vi "StaticCalibration3.vi"(0 "SENSOR":T1, 11 "error in (no error)":errorcluster caption="错误输入（无错误）") -> (2 "T1(%)":dbl, 3 "T2(%)":dbl, 4 "Vres":dbl, 6 "Angle out":dbl, 8 "Vres_FD":i32, 10 "OK":bool, 13 "P(%)":dbl, 14 "S(%)":dbl, 15 "error out":errorcluster caption="错误输出")   [LabVIEW 2020]
doc: "该模板用于创建子VI。"
uses:
  <userlib>/DAQNavi Polymorphic VI/create/DAQNavi Create Channel.vi
  <userlib>/DAQNavi Polymorphic VI/create/DAQNavi Create Channel(CI-PulseWidth).vi
  <userlib>/DAQNavi Polymorphic VI/read/DAQNavi Read.vi
  <userlib>/DAQNavi Polymorphic VI/read/DAQNavi Read (Counter Pulse Width 1Chan 1Samp).vi
  <userlib>/_MGI/1D Array/MGI Average.vi
  <userlib>/_MGI/1D Array/MGI Average/MGI Average (DBL[]).vi
  <userlib>/DAQNavi Polymorphic VI/configure/task/DAQNavi Clear Task.vi
  Global_Variable/Global.vi
  <vilib>/Comparison/Less/Less Functor/Less Functor.lvclass
  <userlib>/Hella PGI/Hella PGI.lvlib
panel:
  out "T2ROC_1+T2ROC_2":i32
  out "T1ROC_1+T1ROC_2":i32
  out "PROC_1":i32
  out "T2ROC_1":i32
  out "T1ROC_1":i32
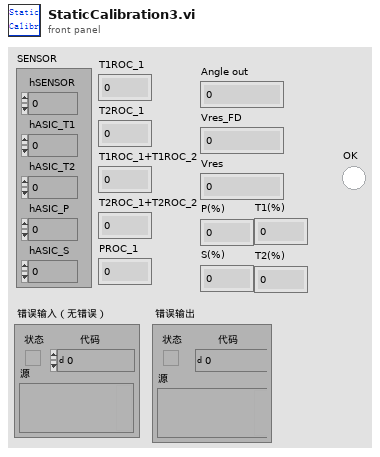
[diagram p1: front panel]
types:
  T1 = cluster{"hSENSOR":i32, "hASIC_T1":i32, "hASIC_T2":i32, "hASIC_P":i32, "hASIC_S":i32}
  T2 = cluster{"主信号":cluster{"单位":string, "下限":dbl, "上限":dbl}, "副信号":cluster{"单位":string, "下限":dbl, "上限":dbl}, "主副和":cluster{"单位":string, "下限":dbl, "上限":dbl}, "主副差":cluster{"单位":string, "下限":dbl, "上限":dbl}, "Vres":cluster{"单位":string, "下限":dbl, "上限":dbl}}
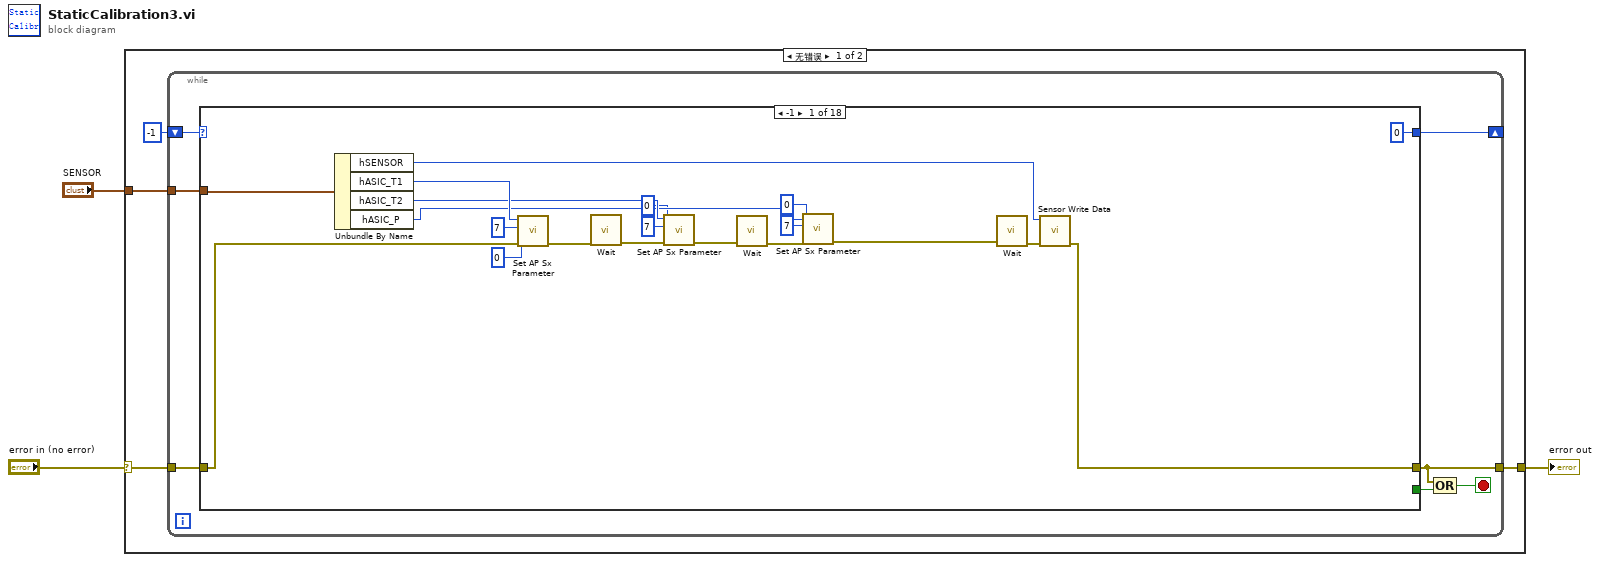
[diagram p0: block diagram]
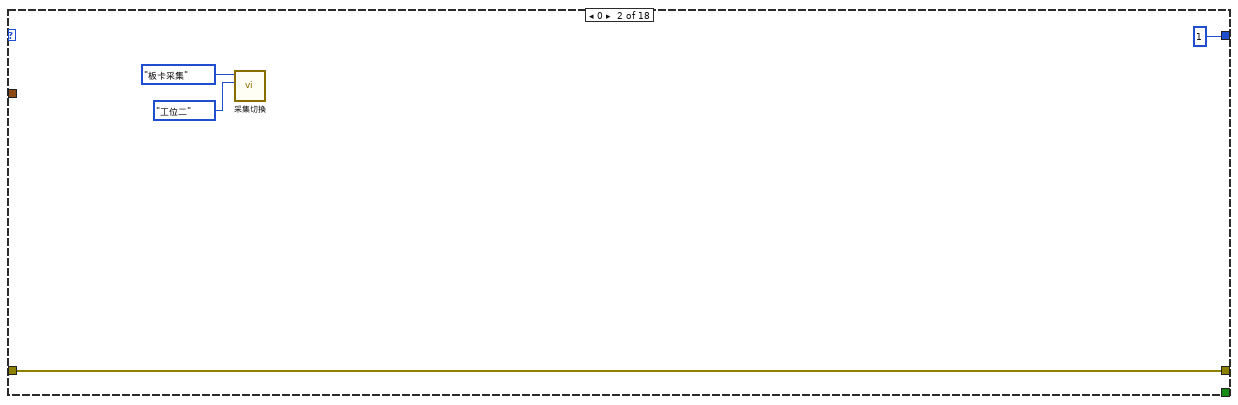
[diagram p2: hidden frame]
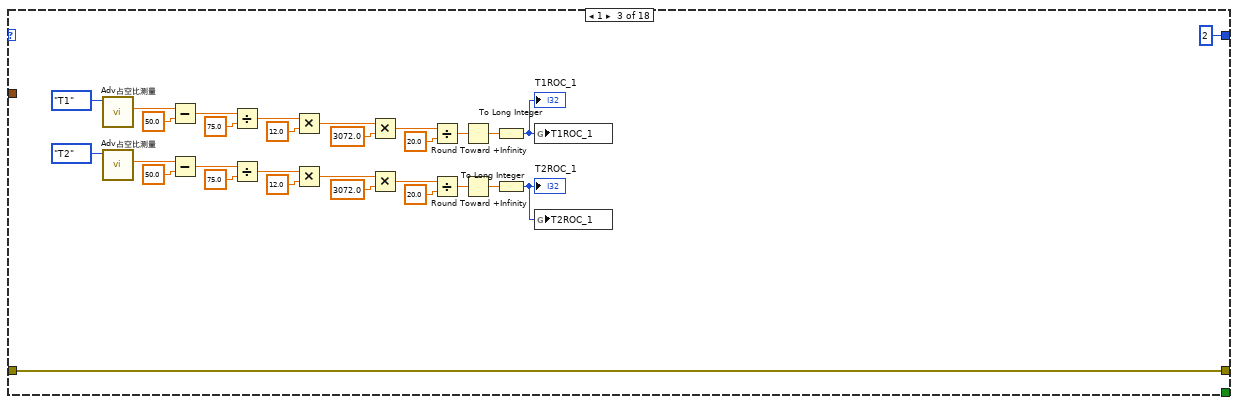
[diagram p3: hidden frame]
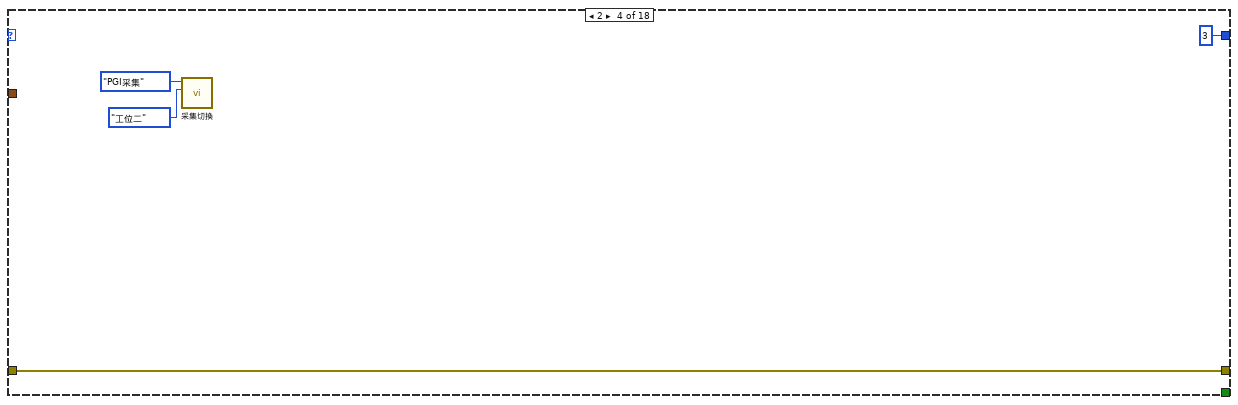
[diagram p4: hidden frame]
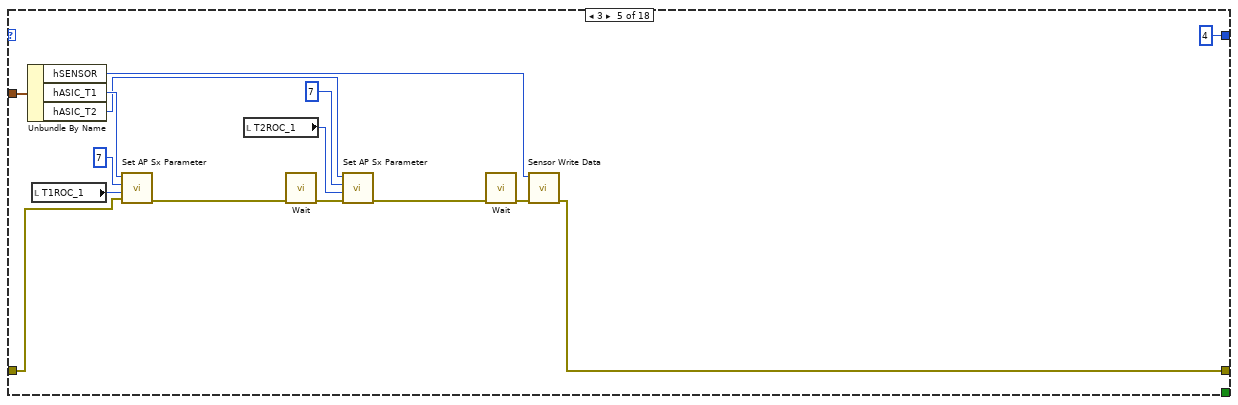
[diagram p5: hidden frame]
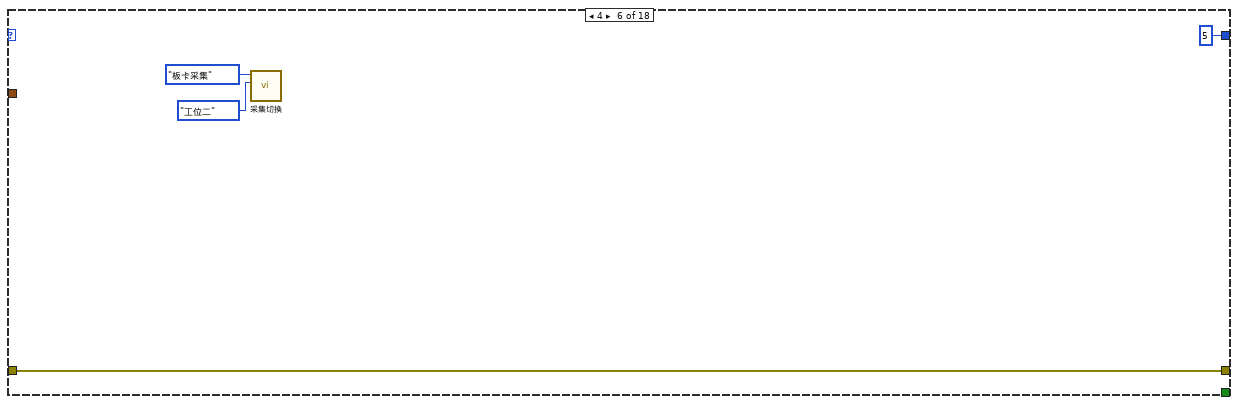
[diagram p6: hidden frame]
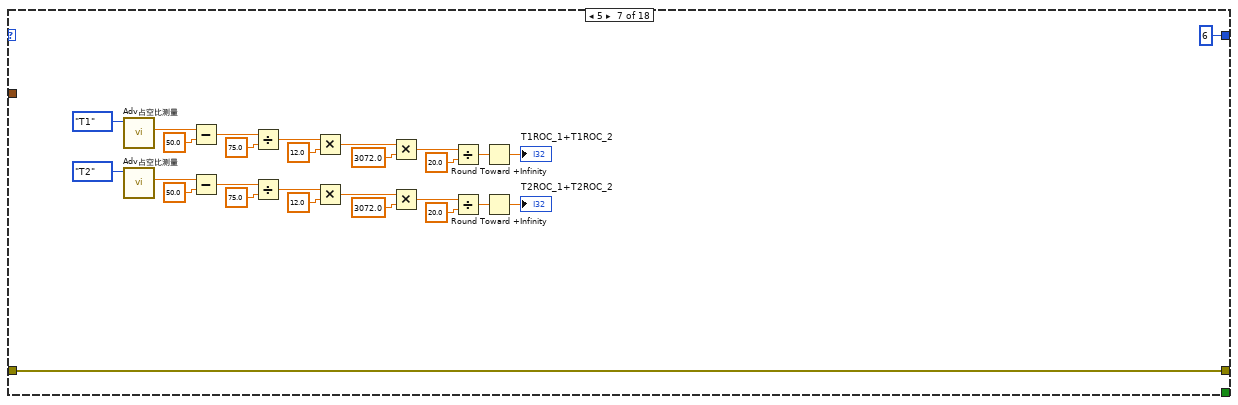
[diagram p7: hidden frame]
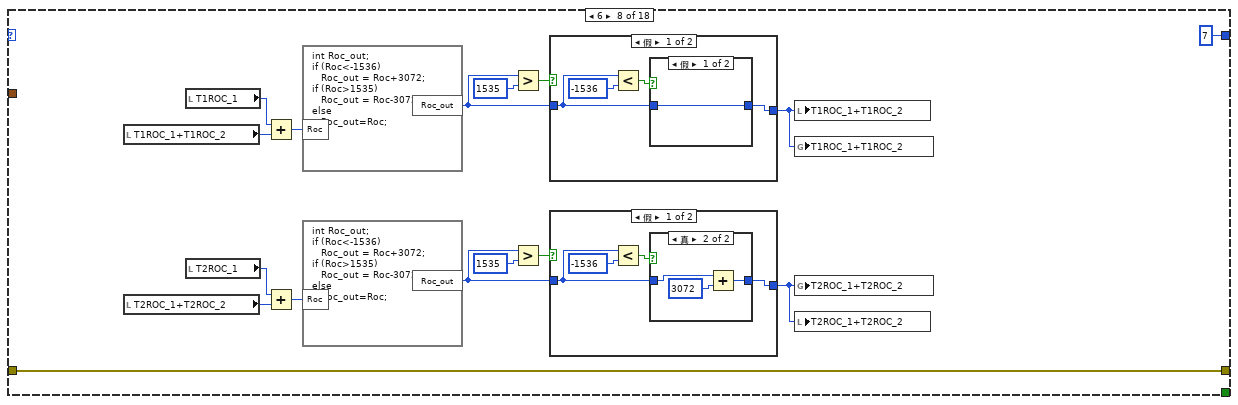
[diagram p8: hidden frame]
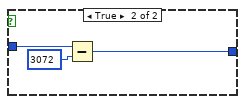
[diagram p10: hidden frame]
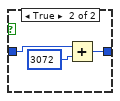
[diagram p11: hidden frame]
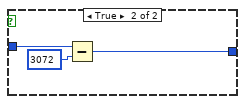
[diagram p12: hidden frame]
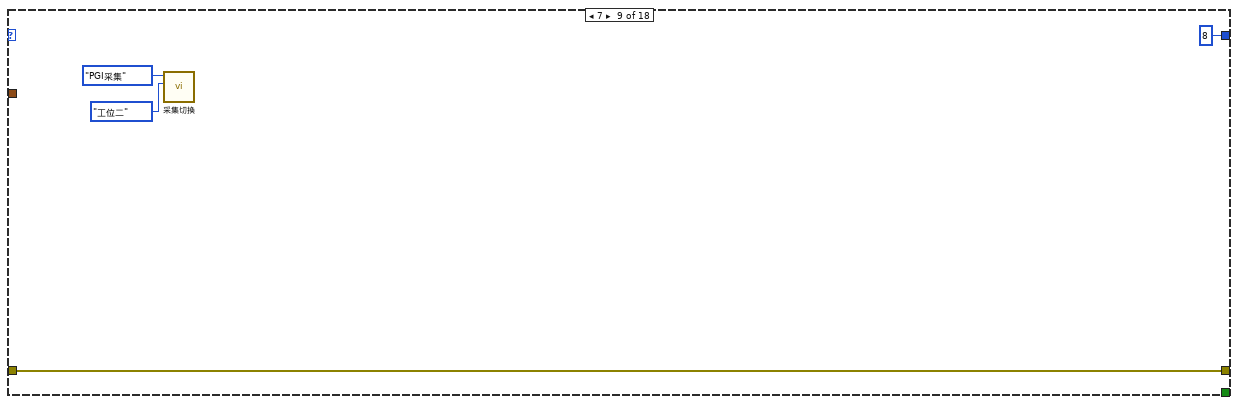
[diagram p13: hidden frame]
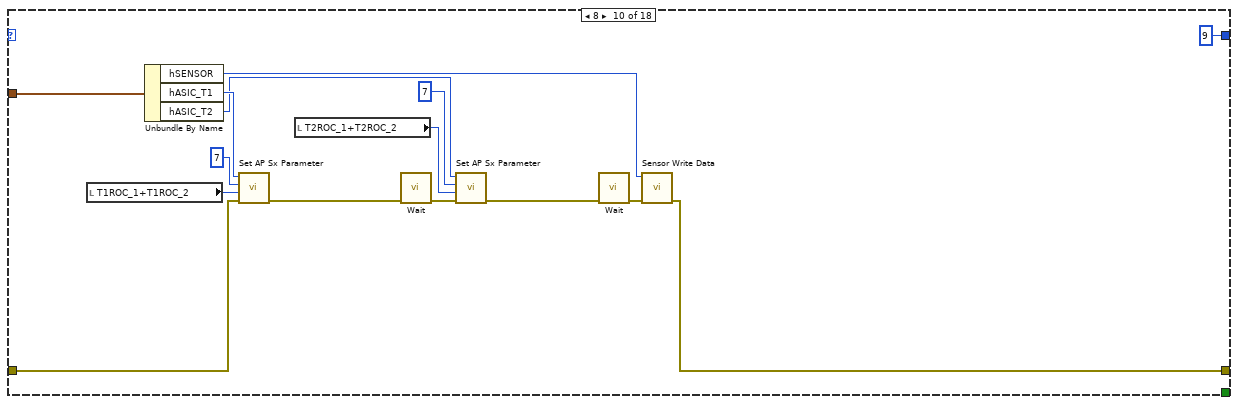
[diagram p14: hidden frame]
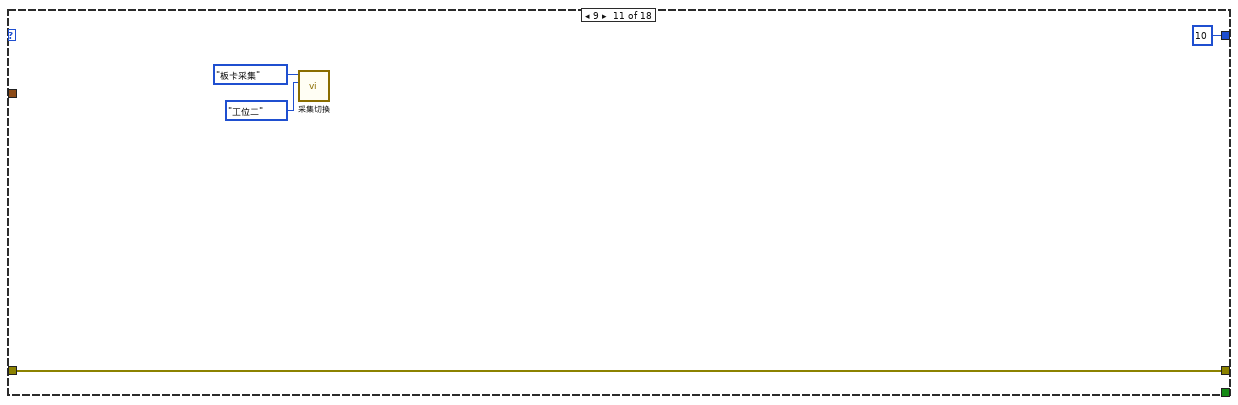
[diagram p15: hidden frame]
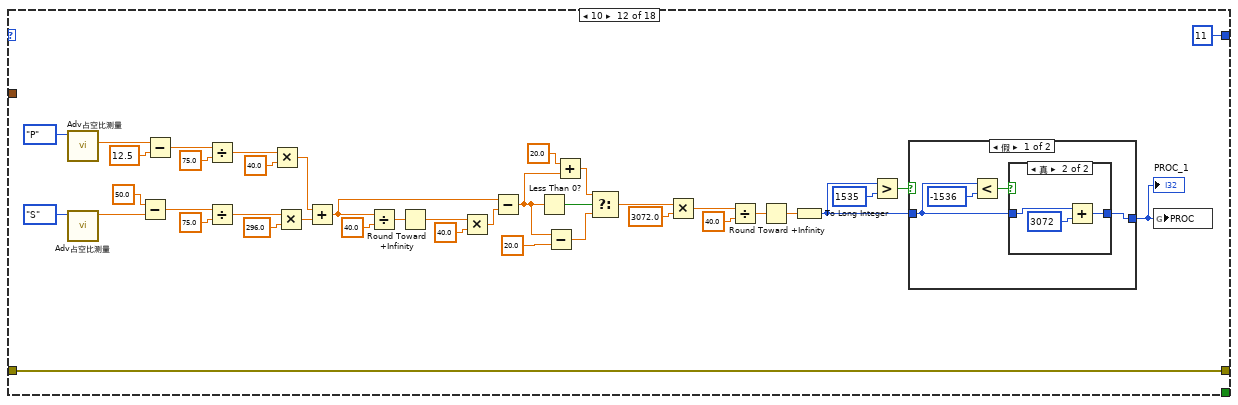
[diagram p16: hidden frame]
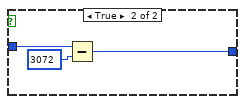
[diagram p18: hidden frame]
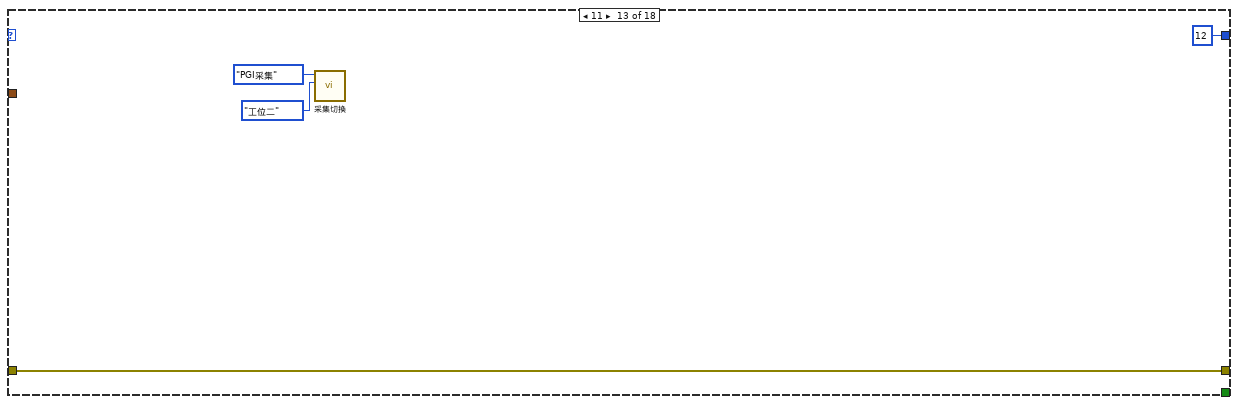
[diagram p19: hidden frame]
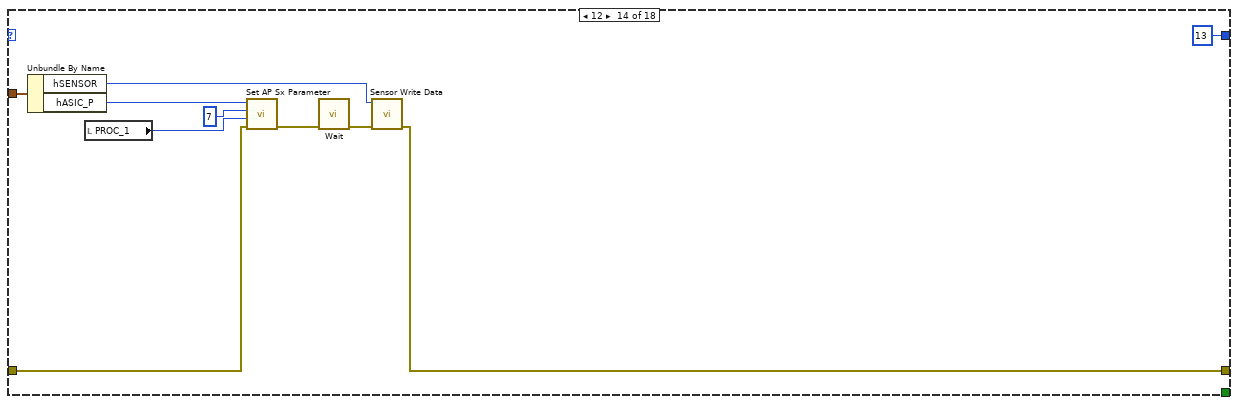
[diagram p20: hidden frame]
diagram:
  n1 = case shown="无错误" "error in (no error)" {
    selector: "error in (no error)" -> [w6 w273]
    tunnel: [w4 w273] -> w2
    tunnel: "SENSOR" -> [w7 _]
    frame No Error {
      n2 = while {
        tunnel: w7 -> [w14]
        tunnel: w6 -> [w13]
        shift-right: [w8] -> _
        shift-left: -1 -> [w12]
        tunnel: [w11] -> w4
        stop <- w10 stop-if-true
        n3 = case shown="-1" w12 {
          tunnel: w14 -> [w18 _ _ _ w85 _ _ _ _ w175 _ _ _ w241 _ _ _ _]
          tunnel: w13 -> [w17 w36 w39 w69 w79 w89 w92 w120 w158 w163 w177 w184 w232 w237 w246 w250 w264 w272]
          selector: w12 -> [_ _ _ _ _ _ _ _ _ _ _ _ _ _ _ _ _ w270]
          tunnel: [w16 w36 w39 w69 w73 w89 w92 w120 w158 w162 w177 w184 w232 w236 w246 w250 w264 w272] -> w11
          tunnel: [_ _ _ _ _ _ _ _ _ _ _ _ _ _ _ _ _ TRUE] -> w9
          tunnel: [0 1 2 3 4 5 6 7 8 9 10 11 12 13 14 15 16 w270] -> w8
          frame -1 {
            n4 = Unbundle By Name(w18) -> ("hSENSOR"=w31:i32, "hASIC_T1"=w25:i32, "hASIC_T2"=w24:i32, "hASIC_P"=w23:i32)
            n5 = call <userlib>:"Set AP Sx Parameter.vi"("error in (no error)"=w17, "para2"=0, "asicBitsName"=7, "asicHandle"=w25) -> ("error out"=w29:errorcluster)  [unwired: 6 in, 1 out]
            n6 = call "Wait.vi"("error in (no error)"=w29) -> ("error out"=w30:errorcluster)  [unwired: 6 in]
            n7 = call <userlib>:"Set AP Sx Parameter.vi"("error in (no error)"=w30, "para2"=0, "asicBitsName"=7, "asicHandle"=w24) -> ("error out"=w28:errorcluster)  [unwired: 6 in, 1 out]
            n8 = call "Wait.vi"("error in (no error)"=w28) -> ("error out"=w27:errorcluster)  [unwired: 6 in]
            n9 = call <userlib>:"Set AP Sx Parameter.vi"("error in (no error)"=w27, "para2"=0, "asicBitsName"=7, "asicHandle"=w23) -> ("error out"=w26:errorcluster)  [unwired: 6 in, 1 out]
            n10 = call "Wait.vi"("error in (no error)"=w26) -> ("error out"=w34:errorcluster)  [unwired: 6 in]
            n11 = call <userlib>:"Sensor Write Data.vi"("error in (no error)"=w34, "sensorHandle"=w31) -> ("error out"=w16:errorcluster)  [unwired: 7 in, 2 out]
          }
          frame 0 {
            n12 = call "采集切换.vi"("工位"=enum16{"工位一", "工位二"}."工位二", "采集方式"=enum16{"板卡采集", "PGI采集"}."板卡采集") -> ()  [unwired: 10 in]
          }
          frame 1 {
            n13 = call "Adv占空比测量.vi"("通道"=enum16{"T1", "T2", "P", "S"}."T1") -> ("占空比2"=w43:dbl)  [unwired: 7 in, 2 out]
            n14 = call "Adv占空比测量.vi"("通道"=enum16{"T1", "T2", "P", "S"}."T2") -> ("占空比2"=w41:dbl)  [unwired: 7 in, 2 out]
            n15 = Subtract(x=w43, y=50.0) -> (x-y=w67:dbl)
            n16 = Subtract(x=w41, y=50.0) -> (x-y=w52:dbl)
            n17 = Divide(x=w67, y=75.0) -> (x/y=w65:dbl)
            n18 = Divide(x=w52, y=75.0) -> (x/y=w54:dbl)
            n19 = Multiply(x=w65, y=12.0) -> (x*y=w63:dbl)
            n20 = Multiply(x=w54, y=12.0) -> (x*y=w56:dbl)
            n21 = Multiply(x=w63, y=3072.0) -> (x*y=w61:dbl)
            n22 = Multiply(x=w56, y=3072.0) -> (x*y=w58:dbl)
            n23 = Divide(x=w61, y=20.0) -> (x/y=w50:dbl)
            n24 = Divide(x=w58, y=20.0) -> (x/y=w49:dbl)
            n25 = Round Toward +Infinity(x=w50) -> (ceil(x): smallest int >= x=w48:dbl)
            n26 = Round Toward +Infinity(x=w49) -> (ceil(x): smallest int >= x=w47:dbl)
            n27 = To Long Integer(number=w48) -> (32bit integer=w45:i32)
            "T1ROC_1" <- w45
            n28 = To Long Integer(number=w47) -> (32bit integer=w46:i32)
            "T2ROC_1" <- w46
            n29 = global write "Global.vi" "T1ROC_1"(w45) -> ()
            n30 = global write "Global.vi" "T2ROC_1"(w46) -> ()
          }
          frame 2 {
            n31 = call "采集切换.vi"("工位"=enum16{"工位一", "工位二"}."工位二", "采集方式"=enum16{"板卡采集", "PGI采集"}."PGI采集") -> ()  [unwired: 10 in]
          }
          frame 3 {
            n32 = Unbundle By Name(w85) -> ("hSENSOR"=w82:i32, "hASIC_T1"=w84:i32, "hASIC_T2"=w83:i32)
            n33 = local read "T1ROC_1"() -> (w86:i32)
            n34 = call <userlib>:"Set AP Sx Parameter.vi"("error in (no error)"=w79, "para2"=w86, "asicBitsName"=7, "asicHandle"=w84) -> ("error out"=w78:errorcluster)  [unwired: 6 in, 1 out]
            n35 = local read "T2ROC_1"() -> (w87:i32)
            n36 = call "Wait.vi"("error in (no error)"=w78) -> ("error out"=w77:errorcluster)  [unwired: 6 in]
            n37 = call <userlib>:"Set AP Sx Parameter.vi"("error in (no error)"=w77, "para2"=w87, "asicBitsName"=7, "asicHandle"=w83) -> ("error out"=w76:errorcluster)  [unwired: 6 in, 1 out]
            n38 = call "Wait.vi"("error in (no error)"=w76) -> ("error out"=w75:errorcluster)  [unwired: 6 in]
            n39 = call <userlib>:"Sensor Write Data.vi"("error in (no error)"=w75, "sensorHandle"=w82) -> ("error out"=w73:errorcluster)  [unwired: 7 in, 2 out]
          }
          frame 4 {
            n40 = call "采集切换.vi"("工位"=enum16{"工位一", "工位二"}."工位二", "采集方式"=enum16{"板卡采集", "PGI采集"}."板卡采集") -> ()  [unwired: 10 in]
          }
          frame 5 {
            n41 = call "Adv占空比测量.vi"("通道"=enum16{"T1", "T2", "P", "S"}."T1") -> ("占空比2"=w95:dbl)  [unwired: 7 in, 2 out]
            n42 = call "Adv占空比测量.vi"("通道"=enum16{"T1", "T2", "P", "S"}."T2") -> ("占空比2"=w94:dbl)  [unwired: 7 in, 2 out]
            n43 = Subtract(x=w95, y=50.0) -> (x-y=w112:dbl)
            n44 = Subtract(x=w94, y=50.0) -> (x-y=w119:dbl)
            n45 = Divide(x=w112, y=75.0) -> (x/y=w113:dbl)
            n46 = Divide(x=w119, y=75.0) -> (x/y=w118:dbl)
            n47 = Multiply(x=w113, y=12.0) -> (x*y=w114:dbl)
            n48 = Multiply(x=w118, y=12.0) -> (x*y=w117:dbl)
            n49 = Multiply(x=w114, y=3072.0) -> (x*y=w115:dbl)
            n50 = Multiply(x=w117, y=3072.0) -> (x*y=w116:dbl)
            n51 = Divide(x=w115, y=20.0) -> (x/y=w111:dbl)
            n52 = Divide(x=w116, y=20.0) -> (x/y=w110:dbl)
            n53 = Round Toward +Infinity(x=w111) -> (ceil(x): smallest int >= x=→"T1ROC_1+T1ROC_2":dbl)
            n54 = Round Toward +Infinity(x=w110) -> (ceil(x): smallest int >= x=→"T2ROC_1+T2ROC_2":dbl)
          }
          frame 6 {
            n55 = local read "T1ROC_1+T1ROC_2"() -> (w125:i32)
            n56 = local read "T2ROC_1+T2ROC_2"() -> (w124:i32)
            n57 = local read "T1ROC_1"() -> (w133:i32)
            n58 = local read "T2ROC_1"() -> (w132:i32)
            n59 = Add(x=w133, y=w125) -> (x+y=w135:i32)
            n60 = Add(x=w132, y=w124) -> (x+y=w134:i32)
            n61 = formula code="int Roc_out;\nif (Roc<-1536)\n   Roc_out = Roc+3072;\nif (Roc>1535)\n   Roc_out = Roc-3072;\nelse\n   Roc_out=Roc;"("Roc"=w135) -> ("Roc_out"=w129:i32)
            n62 = formula code="int Roc_out;\nif (Roc<-1536)\n   Roc_out = Roc+3072;\nif (Roc>1535)\n   Roc_out = Roc-3072;\nelse\n   Roc_out=Roc;"("Roc"=w134) -> ("Roc_out"=w126:i32)
            n63 = Greater?(x=w129, y=1535) -> (0:w130:bool)
            n64 = Greater?(x=w126, y=1535) -> (0:w127:bool)
            n65 = case shown="假" w130 {
              tunnel: w129 -> [w148 w156]
              tunnel: [w147 w155] -> w123
              frame False {
                n66 = Less?(x=w148, y=-1536) -> (x < y?=w149:bool)
                n67 = case shown="假" w149 {
                  tunnel: w148 -> [w151 w154]
                  tunnel: [w151 w152] -> w147
                  frame False {
                  }
                  frame True {
                    n68 = Add(x=w154, y=3072) -> (x+y=w152:i32)
                  }
                }
              }
              frame True {
                n69 = Subtract(x=w156, y=3072) -> (x-y=w155:i32)
              }
            }
            n70 = case shown="假" w127 {
              tunnel: w126 -> [w137 w145]
              tunnel: [w136 w144] -> w122
              frame False {
                n71 = Less?(x=w137, y=-1536) -> (x < y?=w138:bool)
                n72 = case shown="真" w138 {
                  tunnel: w137 -> [w140 w143]
                  tunnel: [w140 w141] -> w136
                  frame False {
                  }
                  frame True {
                    n73 = Add(x=w143, y=3072) -> (x+y=w141:i32)
                  }
                }
              }
              frame True {
                n74 = Subtract(x=w145, y=3072) -> (x-y=w144:i32)
              }
            }
            n75 = local write "T1ROC_1+T1ROC_2"(w123) -> ()
            n76 = global write "Global.vi" "T1ROC_1+T1ROC_2"(w123) -> ()
            n77 = global write "Global.vi" "T2ROC_1+T2ROC_2"(w122) -> ()
            n78 = local write "T2ROC_1+T2ROC_2"(w122) -> ()
          }
          frame 7 {
            n79 = call "采集切换.vi"("工位"=enum16{"工位一", "工位二"}."工位二", "采集方式"=enum16{"板卡采集", "PGI采集"}."PGI采集") -> ()  [unwired: 10 in]
          }
          frame 8 {
            n80 = local read "T1ROC_1+T1ROC_2"() -> (w171:i32)
            n81 = Unbundle By Name(w175) -> ("hSENSOR"=w172:i32, "hASIC_T1"=w174:i32, "hASIC_T2"=w173:i32)
            n82 = call <userlib>:"Set AP Sx Parameter.vi"("error in (no error)"=w163, "para2"=w171, "asicBitsName"=7, "asicHandle"=w174) -> ("error out"=w168:errorcluster)  [unwired: 6 in, 1 out]
            n83 = local read "T2ROC_1+T2ROC_2"() -> (w176:i32)
            n84 = call "Wait.vi"("error in (no error)"=w168) -> ("error out"=w167:errorcluster)  [unwired: 6 in]
            n85 = call <userlib>:"Set AP Sx Parameter.vi"("error in (no error)"=w167, "para2"=w176, "asicBitsName"=7, "asicHandle"=w173) -> ("error out"=w166:errorcluster)  [unwired: 6 in, 1 out]
            n86 = call "Wait.vi"("error in (no error)"=w166) -> ("error out"=w165:errorcluster)  [unwired: 6 in]
            n87 = call <userlib>:"Sensor Write Data.vi"("error in (no error)"=w165, "sensorHandle"=w172) -> ("error out"=w162:errorcluster)  [unwired: 7 in, 2 out]
          }
          frame 9 {
            n88 = call "采集切换.vi"("工位"=enum16{"工位一", "工位二"}."工位二", "采集方式"=enum16{"板卡采集", "PGI采集"}."板卡采集") -> ()  [unwired: 10 in]
          }
          frame 10 {
            n89 = call "Adv占空比测量.vi"("通道"=enum16{"T1", "T2", "P", "S"}."P") -> ("占空比2"=w189:dbl)  [unwired: 7 in, 2 out]
            n90 = call "Adv占空比测量.vi"("通道"=enum16{"T1", "T2", "P", "S"}."S") -> ("占空比1"=w188:dbl)  [unwired: 7 in, 2 out]
            n91 = Subtract(x=50.0, y=w188) -> (x-y=w213:dbl)
            n92 = Subtract(x=w189, y=12.5) -> (x-y=w219:dbl)
            n93 = Divide(x=w219, y=75.0) -> (x/y=w217:dbl)
            n94 = Divide(x=w213, y=75.0) -> (x/y=w211:dbl)
            n95 = Multiply(x=w217, y=40.0) -> (x*y=w215:dbl)
            n96 = Multiply(x=w211, y=296.0) -> (x*y=w209:dbl)
            n97 = Add(x=w215, y=w209) -> (x+y=w203:dbl)
            n98 = Divide(x=w203, y=40.0) -> (x/y=w207:dbl)
            n99 = Round Toward +Infinity(x=w207) -> (ceil(x): smallest int >= x=w205:dbl)
            n100 = Multiply(x=w205, y=40.0) -> (x*y=w204:dbl)
            n101 = Subtract(x=w203, y=w204) -> (x-y=w183:dbl)
            n102 = Less Than 0?(x=w183) -> (x < 0?=w200:bool)
            n103 = Subtract(x=w183, y=20.0) -> (x-y=w181:dbl)
            n104 = Add(x=20.0, y=w183) -> (x+y=w201:dbl)
            n105 = Select(t=w201, s=w200, f=w181) -> (s? t:f=w199:dbl)
            n106 = Multiply(x=w199, y=3072.0) -> (x*y=w197:dbl)
            n107 = Divide(x=w197, y=40.0) -> (x/y=w192:dbl)
            n108 = Round Toward +Infinity(x=w192) -> (ceil(x): smallest int >= x=w191:dbl)
            n109 = To Long Integer(number=w191) -> (32bit integer=w195:i32)
            n110 = Greater?(x=w195, y=1535) -> (0:w193:bool)
            n111 = case shown="假" w193 {
              tunnel: w195 -> [w222 w230]
              tunnel: [w221 w229] -> w190
              frame False {
                n112 = Less?(x=w222, y=-1536) -> (x < y?=w223:bool)
                n113 = case shown="真" w223 {
                  tunnel: w222 -> [w225 w228]
                  tunnel: [w225 w226] -> w221
                  frame False {
                  }
                  frame True {
                    n114 = Add(x=w228, y=3072) -> (x+y=w226:i32)
                  }
                }
              }
              frame True {
                n115 = Subtract(x=w230, y=3072) -> (x-y=w229:i32)
              }
            }
            "PROC_1" <- w190
            n116 = global write "Global.vi" "PROC"(w190) -> ()
          }
          frame 11 {
            n117 = call "采集切换.vi"("工位"=enum16{"工位一", "工位二"}."工位二", "采集方式"=enum16{"板卡采集", "PGI采集"}."PGI采集") -> ()  [unwired: 10 in]
          }
          frame 12 {
            n118 = Unbundle By Name(w241) -> ("hSENSOR"=w240:i32, "hASIC_P"=w239:i32)
            n119 = local read "PROC_1"() -> (w243:i32)
            n120 = call <userlib>:"Set AP Sx Parameter.vi"("error in (no error)"=w237, "para2"=w243, "asicBitsName"=7, "asicHandle"=w239) -> ("error out"=w245:errorcluster)  [unwired: 6 in, 1 out]
            n121 = call "Wait.vi"("error in (no error)"=w245) -> ("error out"=w244:errorcluster)  [unwired: 6 in]
            n122 = call <userlib>:"Sensor Write Data.vi"("error in (no error)"=w244, "sensorHandle"=w240) -> ("error out"=w236:errorcluster)  [unwired: 7 in, 2 out]
          }
          frame 13 {
            n123 = call "采集切换.vi"("工位"=enum16{"工位一", "工位二"}."工位二", "采集方式"=enum16{"板卡采集", "PGI采集"}."板卡采集") -> ()  [unwired: 10 in]
          }
          frame 14 {
            n124 = call "Adv占空比测量.vi"("通道"=enum16{"T1", "T2", "P", "S"}."T2") -> ("占空比2"=→"T2(%)":dbl)  [unwired: 7 in, 2 out]
            n125 = call "Adv占空比测量.vi"("通道"=enum16{"T1", "T2", "P", "S"}."T1") -> ("占空比2"=→"T1(%)":dbl)  [unwired: 7 in, 2 out]
            n126 = call "Adv占空比测量.vi"("通道"=enum16{"T1", "T2", "P", "S"}."P") -> ("占空比2"=w255:dbl)  [unwired: 7 in, 2 out]
            "P(%)" <- w255
            n127 = call "Adv占空比测量.vi"("通道"=enum16{"T1", "T2", "P", "S"}."S") -> ("占空比1"=w252:dbl)  [unwired: 7 in, 2 out]
            "S(%)" <- w252
            n128 = call "Calc_Vres.vi"("S_Data in"=w252, "P_Data in"=w255) -> ("Vres_FD"=→"Vres_FD":i32, "Vres"=→"Vres":dbl, "Angle out"=→"Angle out":dbl)  [unwired: 7 in]
          }
          frame 15 {
            n129 = global read "Global.vi" "静态标定判定"() -> (w266:T2)
            n130 = local read "T1(%)"() -> (w269:dbl)
            n131 = local read "T2(%)"() -> (w268:dbl)
            n132 = local read "Vres"() -> (w267:dbl)
            n133 = call "静态标定判定.vi"("静态标定判定条件"=w266, "Vres"=w267, "T2(%)"=w268, "T1(%)"=w269) -> ("OK？"=→"OK":bool)  [unwired: 7 in]
          }
          frame 16, Default {
          }
        }
        n134 = Compound Arithmetic op=OR ("复合运算")(w11, w9) -> (w10:bool)
      }
    }
    frame Error {
    }
  }
  "error out" <- w2
